vi "fpga_Shot Control.vi"(0 "reclosing setting":T1={"number of reclosing attempts"=1, "dead times [ms]"=[0, 0, 0, 0, 0, 0, 0], "close pulse duration [ms]"=0, "reclaim time [ms]"=0, "enable synchronism check? (F)"=FALSE, "enable lockout reset? (F)"=FALSE, "lockout reset time [ms]"=0} {"number of reclosing attempts" items=["1"=1, "2"=2, "3"=3, "4"=4, "5"=5, "6"=6, "7"=7]}, 2 "reset to ready state? (F)":bool, 7 "shot trip? (F)":bool, 11 "synchronism check pass? (F)":bool) -> (4 "sequence timer active?":bool, 6 "shot count out":u8, 8 "dead state?":bool, 15 "close pulse signal":bool)   [LabVIEW 2013, in "NI_EP_Protection_FPGA.lvlib"]
uses:
  <vilib>/addons/Electrical Power/Protection/NI_EP_Protection_FPGA.lvlib
  <vilib>/addons/Electrical Power/Protection/Reclosing Logic/subVIs/fpga_Recloser Logic Setting.ctl
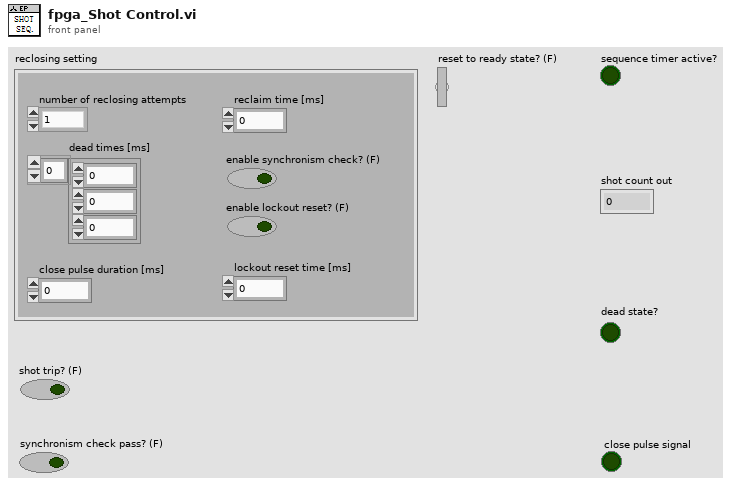
[diagram p1: front panel]
types:
  T1 = typedef "NI_EP_Protection_FPGA.lvlib/fpga_Recloser Logic Setting.ctl" = cluster{"number of reclosing attempts":u8, "dead times [ms]":u32[], "close pulse duration [ms]":u32, "reclaim time [ms]":u32, "enable synchronism check? (F)":bool, "enable lockout reset? (F)":bool, "lockout reset time [ms]":u32}
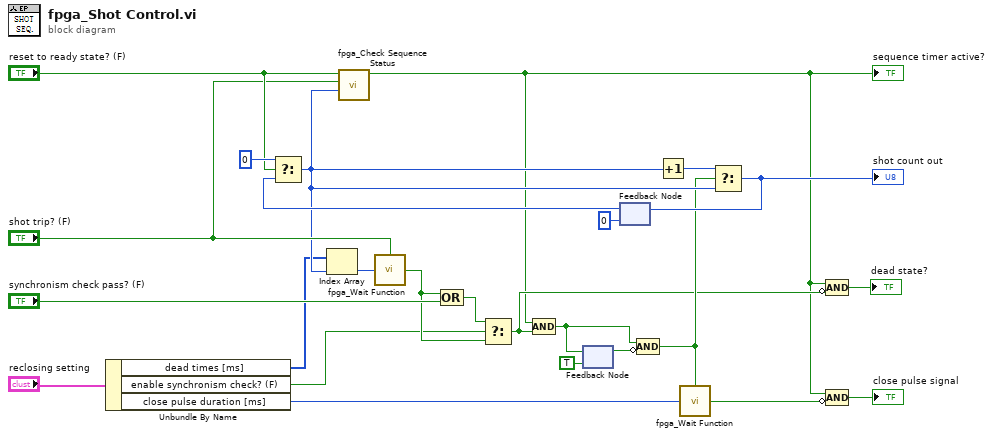
[diagram p0: block diagram]
diagram:
  n1 = Unbundle By Name("reclosing setting") -> ("dead times [ms]"=w7:u32[], "enable synchronism check? (F)"=w6:bool, "close pulse duration [ms]"=w5:u32)
  n2 = feedback #1(TRUE) -> (w21:bool)
  n3 = feedback #2(u8 0) -> (w16:u8)
  n4 = Select(t=u8 0, s="reset to ready state? (F)", f=w16) -> (s? t:f=w13:u8)
  n5 = Index Array(array=w7, index=w13) -> (element=w20:u32)
  n6 = call <vilib>:"fpga_Check Sequence Status.vi"("shot count"=w13, "shot trip? (F)"="shot trip? (F)", "reset to ready state? (F)"="reset to ready state? (F)") -> ("sequence timer active?"=w2:bool)  [unwired: 8 in]
  "sequence timer active?" <- w2
  n7 = call <vilib>:"fpga_Wait Function.vi"("start? (F)"="shot trip? (F)", "timeout (ms)"=w20) -> ("timeout?"=w9:bool)  [unwired: 13 in]
  n8 = Compound Arithmetic op=OR(w9, "synchronism check pass? (F)") -> (w24:bool)
  n9 = Select(t=w24, s=w6, f=w9) -> (s? t:f=w3:bool)
  n10 = Compound Arithmetic op=AND(w2, w3) -> (w8:bool)
  n11 = feedback-in #1(w8) -> ()
  n12 = Compound Arithmetic op=AND(w8, invert w21) -> (w10:bool)
  n13 = Increment(x=w13) -> (x+1=w23:u8)
  n14 = call <vilib>:"fpga_Wait Function.vi"("start? (F)"=w10, "timeout (ms)"=w5) -> ("timeout?"=w12:bool)  [unwired: 13 in]
  n15 = Select(t=w23, s=w10, f=w13) -> (s? t:f=w15:u8)
  "shot count out" <- w15
  n16 = feedback-in #2(w15) -> ()
  n17 = Compound Arithmetic op=AND(w2, invert w3) -> (→"dead state?":bool)
  n18 = Compound Arithmetic op=AND(w2, invert w12) -> (→"close pulse signal":bool)
